vi "Write Scheduled.vi"(1 "scheduled time":timestamp, 2 "element":T1={"Temp. Sensirion"=0.01, "Hum. Sensirion"=0.01, "Temp. Switch Matrix"=0.01, "Hum. Switch Matrix"=0.01, "Temp. Probecard"=0.01, "Hum. Probecard"=0.01} {"Hum. Probecard" format="%#_13g"; "Temp. Probecard" format="%#_13g"; "Hum. Switch Matrix" format="%#_13g"; "Temp. Switch Matrix" format="%#_13g"; "Hum. Sensirion" format="%#_13g"; "Temp. Sensirion" format="%#_13g"}) -> (5 "actual time":timestamp, 7 "channel":T2, 8 "previous element":T1={"Temp. Sensirion"=0.01, "Hum. Sensirion"=0.01, "Temp. Switch Matrix"=0.01, "Hum. Switch Matrix"=0.01, "Temp. Probecard"=0.01, "Hum. Probecard"=0.01} {"Hum. Probecard" format="%#_13g"; "Temp. Probecard" format="%#_13g"; "Hum. Switch Matrix" format="%#_13g"; "Temp. Switch Matrix" format="%#_13g"; "Hum. Sensirion" format="%#_13g"; "Temp. Sensirion" format="%#_13g"})   [LabVIEW 2020, in "Tag-t'data_env.ctl'.lvlib"]
doc: "Writes a value to a Tag channel at the scheduled time."
uses:
  <extravilib>/ChannelInstances/Tag-t'data_env.ctl'.lvlib
  <extravilib>/ChannelInstances/Tag-t'data_env.ctl'/))Channel.ctl
  Desktop/HexDAQ/src/data_env.ctl
  <extravilib>/ChannelInstances/Tag-t'data_env.ctl'/Write With Abort.vi
  <extravilib>/ChannelInstances/Tag-t'data_env.ctl'/Endpoint.vi
  <resource>/ChannelSupport/_ChannelSupport/_ChannelSupport.lvlib
  <resource>/ChannelSupport/_ChannelSupport/GetErrors/FpgaChannelWireNotSupported.xnode
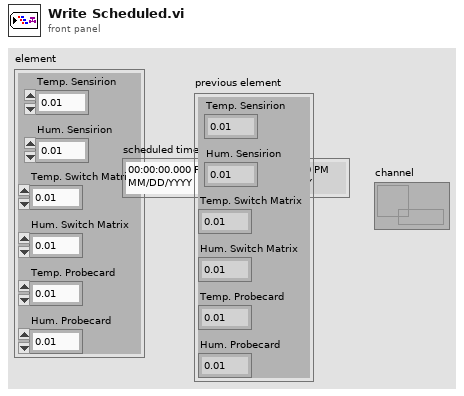
[diagram p1: front panel]
types:
  T1 = typedef "data_env.ctl" = cluster{"Temp. Sensirion":dbl, "Hum. Sensirion":dbl, "Temp. Switch Matrix":dbl, "Hum. Switch Matrix":dbl, "Temp. Probecard":dbl, "Hum. Probecard":dbl}
  T2 = typedef "Tag-t'data_env.ctl'.lvlib/))Channel.ctl" = refnum<queue>
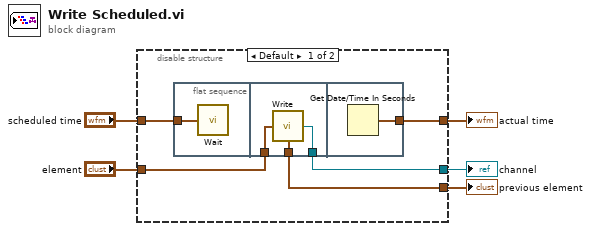
[diagram p0: block diagram]
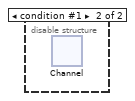
[diagram p2: hidden frame]
diagram:
  n1 = disable-structure shown="Default" {
    disable-tunnel: "scheduled time" -> [w10 _]
    disable-tunnel: [w9 _] -> w4
    disable-tunnel: "element" -> [w8 _]
    disable-tunnel: [w7 _] -> w2
    disable-tunnel: [w6 _] -> w1
    frame condition #0 (active) {
      n2 = flat-sequence {
        tunnel: w10 -> [w11]
        tunnel: w8 -> [w14]
        tunnel: [w13] -> w7
        tunnel: [w12] -> w6
        tunnel: [w15] -> w9
        frame #0 {
          n3 = call <resource>:"Wait.vi"("desired time"=w11) -> ()  [unwired: 2 out]
        }
        frame #1 {
          n4 = call <extravilib>:"Write.vi"("element"=w14) -> ("previous element"=w12:T1, "channel"=w13:T2)
        }
        frame #2 {
          n5 = Get Date/Time In Seconds() -> (seconds since 1Jan1904=w15:timestamp)
        }
      }
    }
    frame condition #1 {
      n6 = xnode "Channel"() -> ()
    }
  }
  "channel" <- w2
  "actual time" <- w4
  "previous element" <- w1
